vi "To VISA Init and Close Enum.vi"(11 "factory init and close behavior":T2) -> (3 "visa init and close behavior":T1)   [LabVIEW 2020, in "VISA Sessions.lvlib" / "Session Factory.lvclass"]
uses:
  Session Factory.lvclass
  Instrument Sessions/ISession Factory/Initialize and Close Session Behavior.ctl
  <vilib>/NI-VISA/VISA gRPC Open Close Behavior.ctl
  Session Factory.lvclass/Session Factory.ctl
  Instrument Sessions/ISession Factory/ISession Factory.lvclass
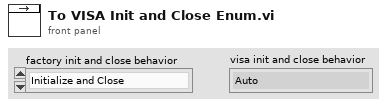
[diagram p1: front panel]
types:
  T1 = typedef "VISA gRPC Open Close Behavior.ctl" = enum16{"Auto", "Initialize and Close", "Attach and Detach", "Initialize and Detach", "Attach and Close"}
  T2 = typedef "Instrument Sessions.lvlib/ISession Factory.lvclass/Initialize and Close Session Behavior.ctl" = enum16{"Initialize and Close", "Attach and Detach", "Initialize and Detach", "Attach and Close"}
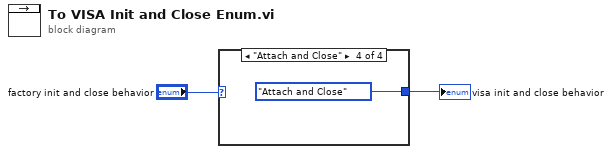
[diagram p0: block diagram]
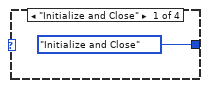
[diagram p2: hidden frame]
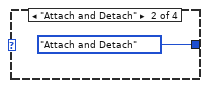
[diagram p3: hidden frame]
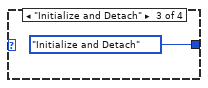
[diagram p4: hidden frame]
diagram:
  n1 = case shown="\"Attach and Close\"" "factory init and close behavior" {
    tunnel: [VISA_gRPC_Open_Close_Behavior."Initialize and Close" ("visa init and close behavior") VISA_gRPC_Open_Close_Behavior."Attach and Detach" ("visa init and close behavior") VISA_gRPC_Open_Close_Behavior."Initialize and Detach" ("visa init and close behavior") VISA_gRPC_Open_Close_Behavior."Attach and Close" ("visa init and close behavior")] -> w1
    frame "Initialize and Close" {
    }
    frame "Attach and Detach" {
    }
    frame "Initialize and Detach" {
    }
    frame "Attach and Close" {
    }
  }
  "visa init and close behavior" <- w1
